vi "FT-IR Max SysLog.vi"(11 "NewVal":T2 {"Max LaserPP" format="%#_5g"; "Max LinCheck" format="%#_5g"; "Max sBeam" format="%#_5g"}) -> (3 "NewVal out":T2 {"Max LaserPP" format="%#_5g"; "Max LinCheck" format="%#_5g"; "Max sBeam" format="%#_5g"})   [LabVIEW 2015, in "FT-IR.lvlib"]
uses:
  FT-IR.lvlib
  Visualisierungs Elemente/Zahlen-Eingabefeld.ctl
  FGV FT-IR Diagnose Aktionen.ctl
  SysLog/SysLog Interface.ctl
  SysLog/SysLog.lvlib
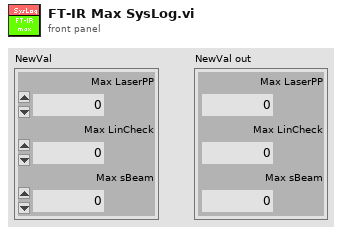
[diagram p1: front panel]
types:
  T1 = typedef "Zahlen-Eingabefeld.ctl" = sgl
  T2 = cluster{"Max LaserPP":T1, "Max LinCheck":T1, "Max sBeam":T1}
  T3 = typedef "FT-IR.lvlib/FGV FT-IR Diagnose Aktionen.ctl" = enum16{"Lesen", "Diagnose Schreiben", "Min Schreiben", "Max Schreiben"}
  T4 = cluster{"LaserPP Max":dbl, "LinCheck Max":dbl, "sBeam Max":dbl}
  T5 = typedef "SysLog.lvlib/SysLog Interface.ctl" = cluster{"FehlermeldungsCode":i32, "ErfolgsmeldungsCode":i32, "ParameterListenString":string, "Anzeige":bool, "SysLogIcon":enum16{"OK", "Warnung", "Fehler"}, "intern":bool}
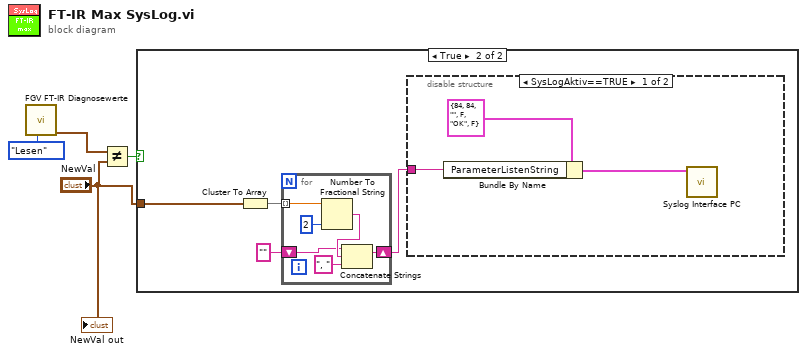
[diagram p0: block diagram]
diagram:
  n1 = call "FGV FT-IR Diagnosewerte.vi"("Aktionen"=FGV_FT-IR_Diagnose_Aktionen."Lesen") -> ("FT-IR MAX"=w2:T4)  [unwired: 5 in, 5 out]
  n2 = Not Equal?(x=w2, y="NewVal") -> (x != y?=w3:bool)
  n3 = case shown="True" w3 {
    tunnel: "NewVal" -> [_ w6]
    frame False {
    }
    frame True {
      n4 = Cluster To Array(cluster=w6) -> (array=w8:T1[])
      n5 = for {
        tunnel: w8 -> [w14] mode=indexing
        shift-right: [w11] -> w5
        shift-left: "" -> [w12]
        n6 = Number To Fractional String(number=w14, precision (6)=i16 2 ("Genauigkeit (6)")) -> (F-format string=w13:string)  [unwired: 2 in]
        n7 = Concatenate Strings(w12, w13, ", " ("String")) -> (w11:string)
      }
      n8 = disable-structure shown="SysLogAktiv==TRUE" {
        disable-tunnel: w5 -> [w16 _]
        frame condition #0 (active) {
          n9 = Bundle By Name(cluster=T5 {"FehlermeldungsCode"=84, "ErfolgsmeldungsCode"=84, "ParameterListenString"="", "Anzeige"=FALSE, "SysLogIcon"=enum."OK", "intern"=FALSE} ("Cluster (in)"), "ParameterListenString"=w16) -> (w15:T5)
          n10 = call "Syslog Interface PC.vi"("Cluster (in)"=w15) -> ()  [unwired: 10 in, 1 out]
        }
        frame condition #1 {
        }
      }
    }
  }
  "NewVal out" <- "NewVal"
